vi "PicoScope3000aExampleStreaming_AdvancedTrig.vi"() -> ()   [LabVIEW 2016]
uses:
  ps3000aWrap.dll
  <vilib>/Waveform/DWDTOps.llb/DWDT Analog to Digital.vi
  PicoScope3000aLib/PicoScope3000aAnalogChannelSettings.ctl
  PicoScope3000aLib/PicoScope3000aDigitalChannelSettings.ctl
panel:
  out "Port 0":digitalwaveform(graph)={"t0"=timestamp(0 s since 1904-01-01), "dt"=1.0000000130088963e-06, "Y"={"transitions"=[], "data"=[]}}
  in  "Port 0 Settings":T1={"Enabled"=FALSE, "Logic Level"=9830} {"Logic Level" items=["1.5V TTL"=9830, "2.5V CMOS"=16383]}
  in  "Auto Trigger (ms)":i32=1000
  in  "Trigger Delay":u32
  in  "Trigger Conditions":T2 {"Condition Logic" items=["AND", "OR", "XOR"]}
  in  "Digital Port  0":T3 {"Direction Channel 7" items=["Don't Care", "Low", "High", "Rising", "Falling"]; "Direction Channel 6" items=["Don't Care", "Low", "High", "Rising", "Falling"]; "Direction Channel 5" items=["Don't Care", "Low", "High", "Rising", "Falling"]; "Direction Channel 4" items=["Don't Care", "Low", "High", "Rising", "Falling"]; "Direction Channel 3" items=["Don't Care", "Low", "High", "Rising", "Falling"]; "Direction Channel 2" items=["Don't Care", "Low", "High", "Rising", "Falling"]; "Direction Channel 1" items=["Don't Care", "Low", "High", "Rising", "Falling"]; "Direction Channel 0" items=["Don't Care", "Low", "High", "Rising", "Falling"]}
  in  "Channel A Trigger Properties":T4={"thresholdUpper"=0, "thresholdUpperHysteresis"=5, "thresholdLower"=0, "thresholdLowerHysteresis"=5, "Threshold Mode"=0, "Direction"=2, "Available"=FALSE} {"Direction" items=["Above / Inside", "Below / Outside", "Rising / Enter", "Falling / Exit", "Rising or Falling / Enter or Exit", "Above Lower", "Below Lower", "Rising Lower", "Falling Lower", "Positive Runt", "Negative Runt"]; "Threshold Mode" items=["Level", "Window"]}
  out "Sample Interval (sec)":dbl format="%#.5p"
  out "AutoStopped":bool
  out "Number of Samples per Capture":i32 format="%#.6p"
  out "Total Samples":u32 format="%#.6p"
  out "TriggeredAt (Total samples)":u32 format="%#.6p"
  out "TriggeredAt (In Buffer)":u32 format="%#.6p"
  out "Triggered":bool
  out "USB 3.0 device on non-USB 3.0 Port":bool
  out "USB Powered":bool
  in  "Channel A Settings":T5={"Enabled"=TRUE, "Coupling"=1, "Range"=6, "Analogue Offset"=0.0, "Bandwidth Limit"=0} {"Bandwidth Limit" items=["Full", "20MHz"]; "Range" items=["10 mV", "20 mV", "50 mV", "100 mV", "200 mV", "500 mV", "1 V", "2 V", "5 V", "10 V", "20 V", "50 V ", "100 V"]; "Coupling" items=["AC", "DC"]}
  in  "Acquisition Settings":T6={"Auto Stop"=TRUE, "Desired Sample Interval"=1, "Pre-trigger Samples"=500000, "Post-trigger Samples"=500000, "Down-Sample Ratio"=1, "Down-Sample Mode"=0, "Overview Buffer Size"=100000, "Time Units"=3, "Four Channel Device?"=FALSE} {"Time Units" items=["Nanoseconds (ns)"=2, "Microseconds (us)"=3, "Milliseconds (ms)"=4, "Seconds (s)"=5]; "Down-Sample Mode" items=["None"=0, "Aggregate"=1, "Decimate"=2, "Average"=4]}
  in  "Apply Settings":bool
  out "Channel A":dbl[](graph)
  in  "stop":bool
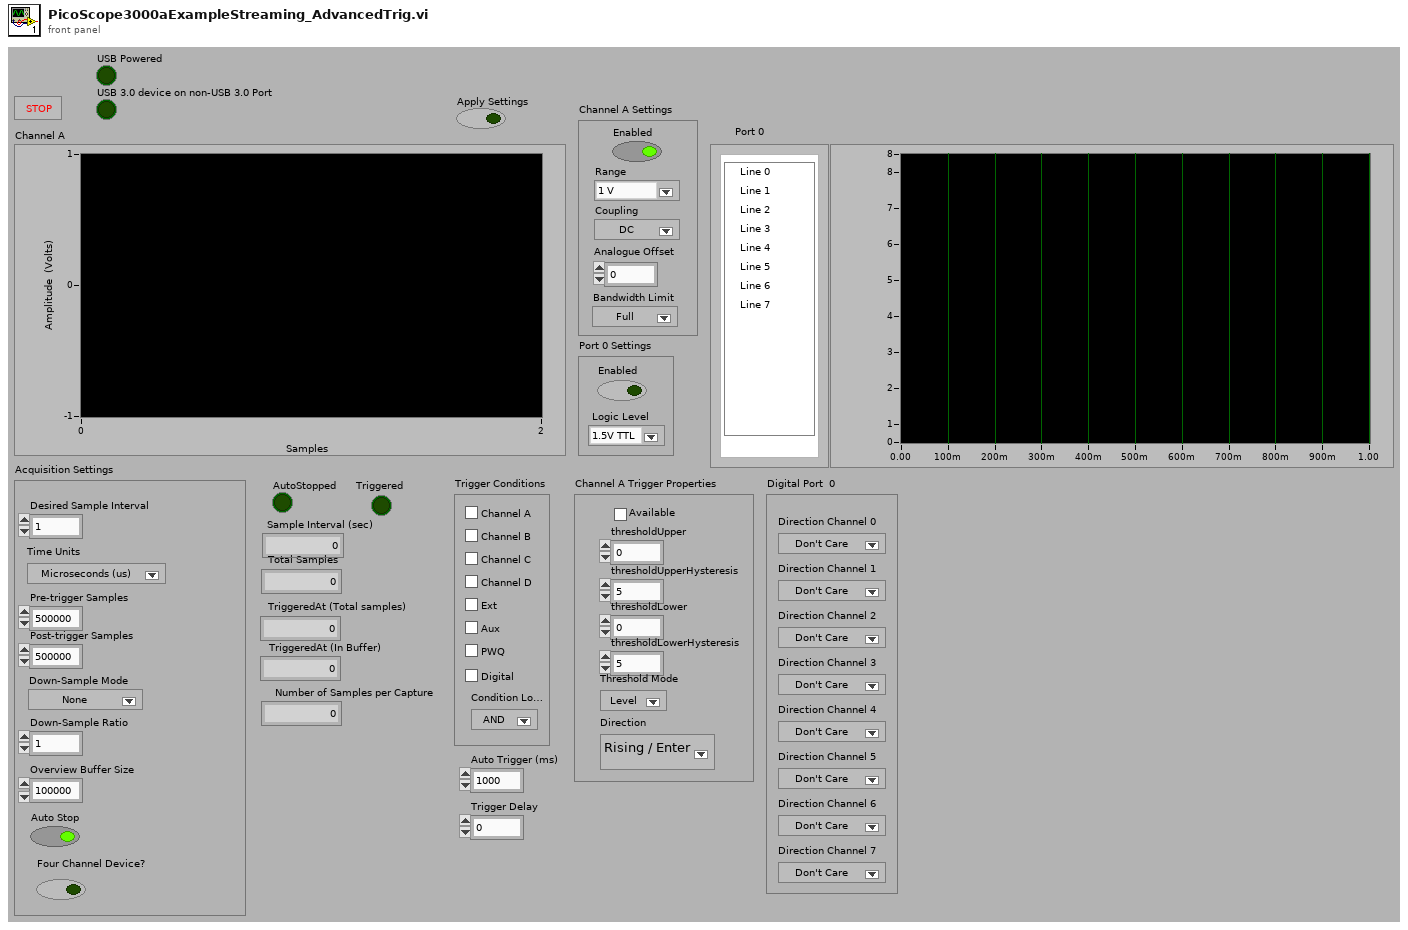
[diagram p1: front panel]
types:
  T1 = typedef "PicoScope3000aDigitalChannelSettings.ctl" = cluster{"Enabled":bool, "Logic Level":i16}
  T2 = cluster{"Channel A":bool, "Channel B":bool, "Channel C":bool, "Channel D":bool, "Aux":bool, "PWQ":bool, "Condition Logic":u16, "Ext":bool, "Digital":bool}
  T3 = cluster{"Direction Channel 0":u16, "Direction Channel 1":u16, "Direction Channel 2":u16, "Direction Channel 3":u16, "Direction Channel 4":u16, "Direction Channel 5":u16, "Direction Channel 6":u16, "Direction Channel 7":u16}
  T4 = cluster{"thresholdUpper":i16, "thresholdUpperHysteresis":u16, "thresholdLower":i16, "thresholdLowerHysteresis":u16, "Threshold Mode":i32, "Direction":i32, "Available":bool}
  T5 = typedef "PicoScope3000aAnalogChannelSettings.ctl" = cluster{"Enabled":bool, "Coupling":u32, "Range":u32, "Analogue Offset":sgl, "Bandwidth Limit":u32}
  T6 = cluster{"Auto Stop":bool, "Desired Sample Interval":u32, "Pre-trigger Samples":u32, "Post-trigger Samples":u32, "Down-Sample Ratio":u32, "Down-Sample Mode":i32, "Overview Buffer Size":u32, "Time Units":u32, "Four Channel Device?":bool}
  T7 = cluster{"Driver Version":string, "USB Version":string, "Hardware":string, "Variant":string, "Batch and Serial":string, "Cal Date":string, "Kernel Version":string, "Digital HW Version":string, "Analogue HW Version":string, "MSO":bool, "Number of channels":i16}
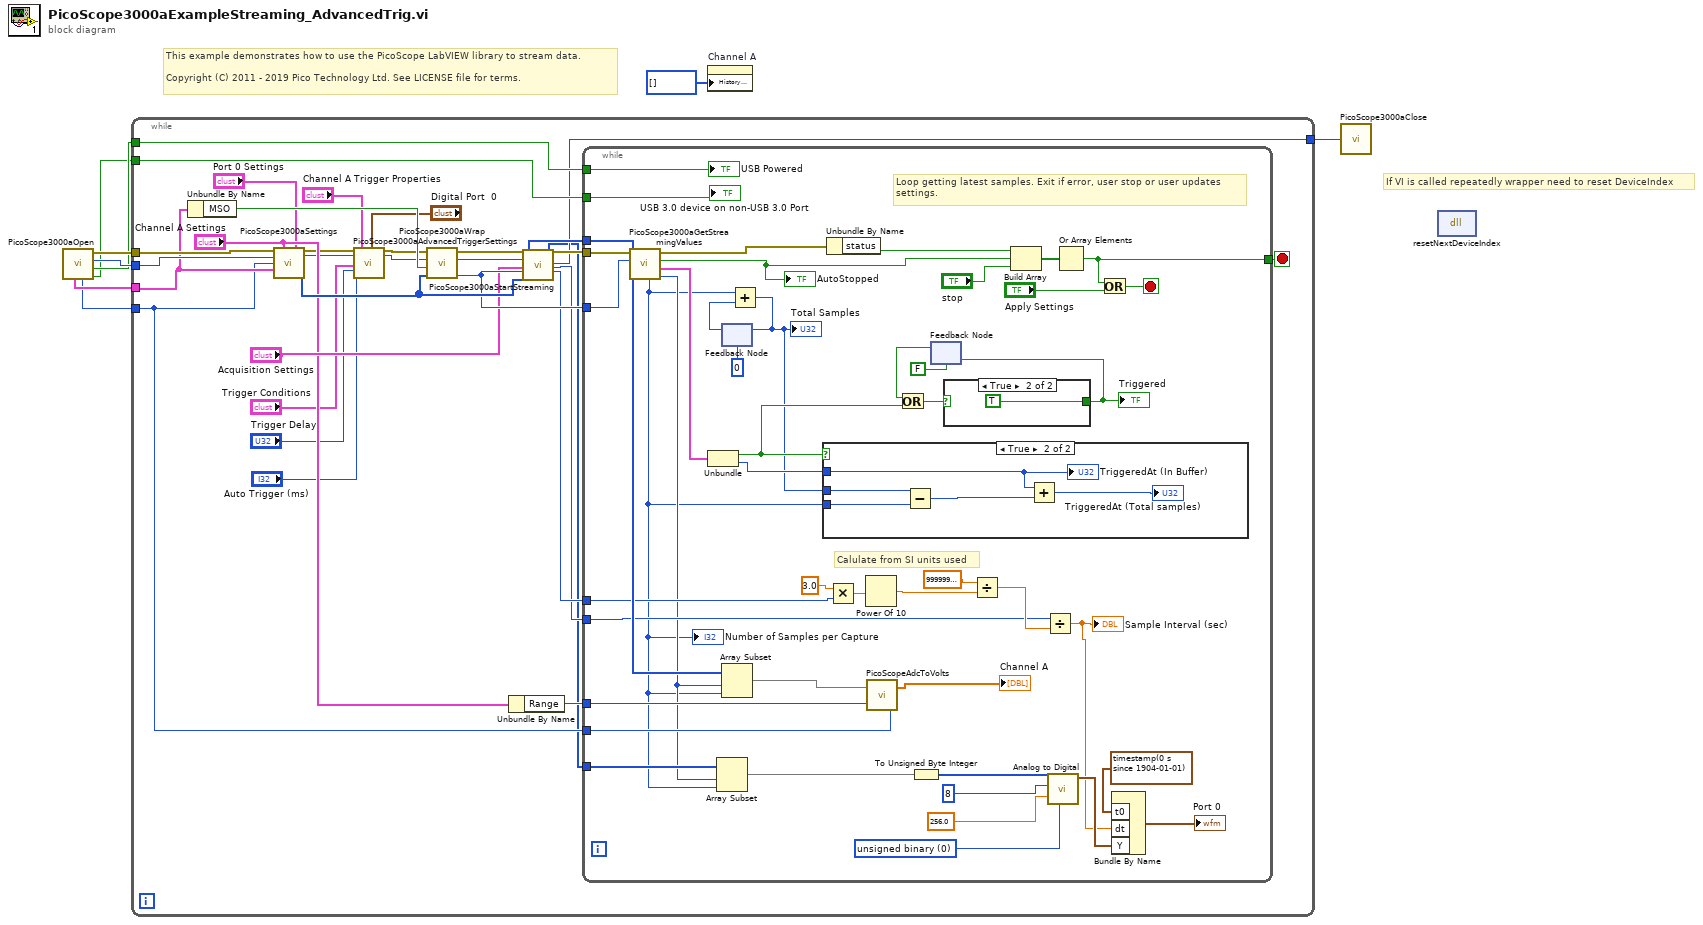
[diagram p0: block diagram]
diagram:
  # "If VI is called repeatedly wrapper need to reset DeviceIndex"
  # "This example demonstrates how to use the PicoScope LabVIEW library to stream data.\n\nCopyright (C) 2011 - 2019 Pico Technology Ltd. See LICENSE file for terms."
  n1 = call "PicoScope3000aOpen.vi"() -> ("USB 3.0 device on non-USB 3.0 Port"=w4:bool, "USB Powered"=w5:bool, "handle"=w6:i16, "error out"=w7:errorcluster, "Max ADC value"=w1:i16, "Device Info"=w2:T7)  [unwired: 6 in]
  n2 = while {
    tunnel: [w29] -> w8
    tunnel: w7 -> [w37]
    tunnel: w6 -> [w38]
    tunnel: w5 -> [w34]
    tunnel: w4 -> [w33]
    tunnel: w2 -> [w26]
    tunnel: w1 -> [w20]
    stop <- w39 stop-if-true
    n3 = Unbundle By Name(w26) -> ("MSO"=w25:bool)
    n4 = call "PicoScope3000aSettings.vi"("error in"=w37, "Channel A Settings"="Channel A Settings", "Port 0 Settings"="Port 0 Settings", "handle in"=w38, "Max_adc"=w20, "Device Info"=w26) -> ("error out"=w19:errorcluster, "handle out"=w17:i16, "Enabled Array"=w30:i16[])  [unwired: 7 in]
    n5 = call "PicoScope3000aAdvancedTriggerSettings.vi"("error in"=w19, "handle in"=w17, "Trigger Conditions"="Trigger Conditions", "Trigger Delay"="Trigger Delay", "Auto Trigger (ms)"="Auto Trigger (ms)", "Channel A Trigger Properties"="Channel A Trigger Properties", "Digital Port  0"="Digital Port  0") -> ("error out"=w18:errorcluster, "handle out"=w16:i16)  [unwired: 11 in]
    n6 = call "PicoScope3000aWrap.vi"("Enabled Array"=w30, "MSO Device?"=w25, "handle in"=w16, "error in (no error)"=w18) -> ("deviceIndex"=w28:u16, "handle out"=w31:i16, "error out"=w32:errorcluster)  [unwired: 1 in]
    n7 = Unbundle By Name("Channel A Settings") -> ("Range"=w22:u32)
    n8 = call "PicoScope3000aStartStreaming.vi"("error in"=w32, "handle in"=w31, "Acquisition Settings"="Acquisition Settings", "deviceIndex"=w28, "Enabled Array"=w30) -> ("Channel A"=w36:i16[], "Port 0 Min"=w9:i16[], "error out"=w35:errorcluster, "handle out"=w29:i16, "Sample Interval"=w23:u32, "sampleIntervalTimeUnits"=w24:i32)  [unwired: 7 in, 10 out]
    n9 = while {
      tunnel: [w75] -> w39
      tunnel: w36 -> [w83]
      tunnel: w35 -> [w81]
      tunnel: w34 -> [w74]
      tunnel: w33 -> [w73]
      tunnel: w28 -> [w80]
      tunnel: w24 -> [w59]
      tunnel: w23 -> [w56]
      tunnel: w22 -> [w54]
      tunnel: w20 -> [w53]
      tunnel: w9 -> [w47]
      stop <- w84 stop-if-true
      w49 = u16 0 items=["unsigned binary", "offset binary", "2's complement"] ("data format (offset binary)")
      # "Loop getting latest samples. Exit if error, user stop or user updates \nsettings."
      # "Calulate from SI units used"
      n10 = call "PicoScope3000aGetStreamingValues.vi"("DeviceIndex"=w80, "error in"=w81) -> ("Start Index"=w46:u32, "Trigger"=w68:cluster{bool, "triggeredAt":u32}, "AutoStopped"=w77:bool, "error out"=w82:errorcluster, "Number of Samples"=w45:i32)  [unwired: 5 in]
      "Number of Samples per Capture" <- w45
      "AutoStopped" <- w77
      n11 = Unbundle(w68) -> (w67:bool, "triggeredAt"=w66:u32)
      n12 = Array Subset(array=w47, index=w46, length=w45) -> (w44:i16[])
      n13 = feedback #1(u32 0) -> (w64:u32)
      n14 = Array Subset(array=w83, index=w46, length=w45) -> (w55:i16[])
      n15 = Add(x=w45, y=w64) -> (x+y=w63:u32)
      "Total Samples" <- w63
      n16 = feedback-in #1(w63) -> ()
      n17 = case shown="True" w67 {
        tunnel: w45 -> [_ w86]
        tunnel: w63 -> [_ w90]
        tunnel: w66 -> [_ w88]
        frame False {
        }
        frame True {
          n18 = Subtract(x=w90, y=w86) -> (x-y=w89:u32)
          n19 = Add(x=w88, y=w89) -> (x+y=→"TriggeredAt (Total samples)":u32)
          "TriggeredAt (In Buffer)" <- w88
        }
      }
      n20 = Unbundle By Name(w82) -> ("status"=w79:bool)
      n21 = Multiply(x=3.0, y=w59) -> (x*y=w60:dbl)
      n22 = Power Of 10(x=w60) -> (10^x=w57:dbl)
      n23 = call "PicoScopeAdcToVolts.vi"("Max_adc"=w53, "Range Index"=w54, "Data"=w55) -> ("Data"=→"Channel A":dbl[])
      n24 = To Unsigned Byte Integer(number=w44) -> (unsigned 8bit integer=w48:u8[])
      n25 = feedback #2(FALSE) -> (w69:bool)
      n26 = Or(x=w69, y=w67) -> (x .or. y?=w71:bool)
      n27 = case shown="True" w71 {
        selector: w71 -> [w91 _]
        tunnel: [w91 TRUE] -> w70
        frame False {
        }
        frame True {
        }
      }
      "Triggered" <- w70
      n28 = feedback-in #2(w70) -> ()
      n29 = Divide(x=sgl 1000000000000000.0 ("y"), y=w57) -> (x/y=w58:dbl)
      n30 = Build Array(w79, w77, "stop") -> (w76:bool[])
      n31 = Divide(x=w56, y=w58) -> (x/y=w40:dbl)
      "Sample Interval (sec)" <- w40
      n32 = call-poly <vilib>:"Analog to Digital.vi"("data format (offset binary)"=w49, "full-scale range (pk-pk)"=256.0, "resolution (16 bit)"=8, "analog waveform"=w48) -> ("digital waveform"=w41:digitalwaveform)  [unwired: 4 in, 3 out]
      n33 = Or Array Elements(Boolean array=w76) -> (logical OR=w75:bool)
      n34 = Or(x=w75, y="Apply Settings") -> (x .or. y?=w84:bool)
      n35 = Bundle By Name("t0"=timestamp(0 s since 1904-01-01), "dt"=w40, "Y"=w41) -> (→"Port 0":digitalwaveform)  [unwired: 1 in]
      "USB Powered" <- w74
      "USB 3.0 device on non-USB 3.0 Port" <- w73
    }
  }
  n36 = property on="Channel A" class="WFChart (strict)"("History Data"=i16[] []) -> ()  [unwired: 2 in, 2 out]
  n37 = call "PicoScope3000aClose.vi"("handle"=w8) -> ()
  n38 = dll-call lib="ps3000aWrap.dll" fn="resetNextDeviceIndex"() -> ()  [unwired: 4 in, 2 out]
